vi "ReadConfigurationFile.vi"(8 "Error in":errorcluster, 11 "Configuration File Path":path) -> (0 "Error out":errorcluster, 3 "App Configuration":T1)   [LabVIEW 2019]
uses:
  #cluster_AppConfiguration.ctl
  <vilib>/Utility/config.llb/Read Key (Path).vi
  <vilib>/Utility/config.llb/NI_LVConfig.lvlib
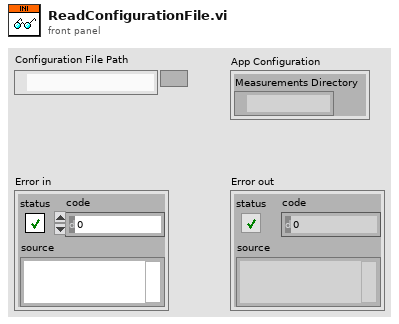
[diagram p1: front panel]
types:
  T1 = typedef "#cluster_AppConfiguration.ctl" = cluster{"Measurements Directory":path}
  T2 = typedef "NI_LVConfig.lvlib/Config Data RefNum.ctl" = refnum<k1>
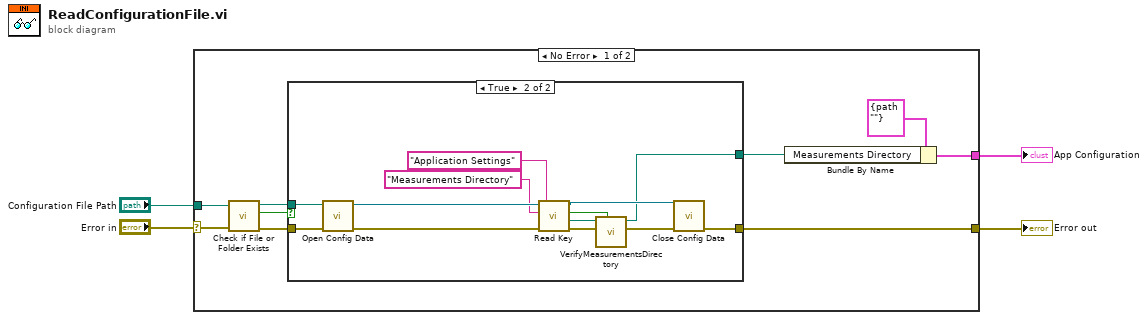
[diagram p0: block diagram]
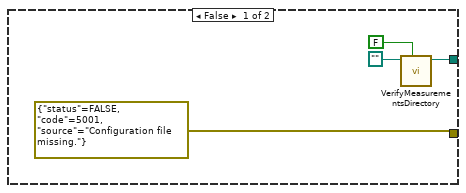
[diagram p2: hidden frame]
diagram:
  n1 = case shown="No Error" "Error in" {
    selector: "Error in" -> [w9 w31]
    tunnel: "Configuration File Path" -> [w13 _]
    tunnel: [w8 w31] -> w2
    tunnel: [w5 _] -> w1
    frame No Error {
      n2 = call <vilib>:"Check if File or Folder Exists.vi"("error in (no error)"=w9, "path"=w13) -> ("error out"=w11:errorcluster, "file or folder exists?"=w12:bool, "dup path"=w10:path)  [unwired: 7 in]
      n3 = case shown="True" w12 {
        tunnel: w11 -> [_ w29]
        tunnel: w10 -> [_ w30]
        tunnel: [errorcluster {"status"=FALSE, "code"=5001, "source"="Configuration file missing."} ("error constant") w24] -> w8
        tunnel: [w16 w18] -> w6
        frame False {
          n4 = call "VerifyMeasurementsDirectory.vi"("Key Found?"=FALSE, "Measurements Directory Path in"=path "") -> ("Measurements Directory Path out"=w16:path)  [unwired: 8 in, 1 out]
        }
        frame True {
          n5 = call <vilib>:"Open Config Data.vi"("error in (no error)"=w29, "configuration file path"=w30) -> ("error out"=w28:errorcluster, "refnum"=w27:T2)  [unwired: 7 in, 1 out]
          n6 = call-poly <vilib>:"Read Key.vi"("section"="Application Settings", "error in (no error)"=w28, "key"="Measurements Directory" ("section"), "refnum"=w27) -> ("error out"=w21:errorcluster, "value"=w23:path, "found?"=w22:bool, "refnum out"=w19:T2)  [unwired: 4 in]
          n7 = call "VerifyMeasurementsDirectory.vi"("Key Found?"=w22, "Error in"=w21, "Measurements Directory Path in"=w23) -> ("Error out"=w20:errorcluster, "Measurements Directory Path out"=w18:path)  [unwired: 7 in]
          n8 = call <vilib>:"Close Config Data.vi"("error in (no error)"=w20, "refnum"=w19) -> ("error out"=w24:errorcluster)  [unwired: 8 in, 1 out]
        }
      }
      n9 = Bundle By Name(cluster=T1 {"Measurements Directory"=path ""} ("App Configuration"), "Measurements Directory"=w6) -> (w5:T1)
    }
    frame Error {
    }
  }
  "Error out" <- w2
  "App Configuration" <- w1
